vi "Create Agent Refnum.vi"(7 "session":T1, 8 "error in (no error)":errorcluster, 11 "LIBSSH2_AGENT*":u64 format="%.0x") -> (0 "error out":errorcluster, 3 "agent":T2)   [LabVIEW 2013, in "libssh2.lvlib"]
uses:
  libssh2.lvlib
  Agent Refnum.ctl
  Session Refnum.ctl
  Agent Refnum Data.ctl
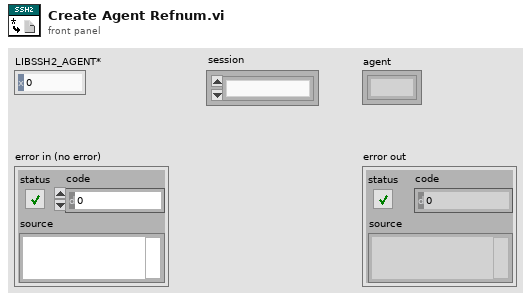
[diagram p1: front panel]
types:
  T1 = typedef "libssh2.lvlib/Session Refnum.ctl" = refnum<k1>
  T2 = typedef "libssh2.lvlib/Agent Refnum.ctl" = refnum<k1>
  T3 = typedef "libssh2.lvlib/Agent Refnum Data.ctl" = cluster{"LIBSSH2_AGENT*":u64, "session":T1}
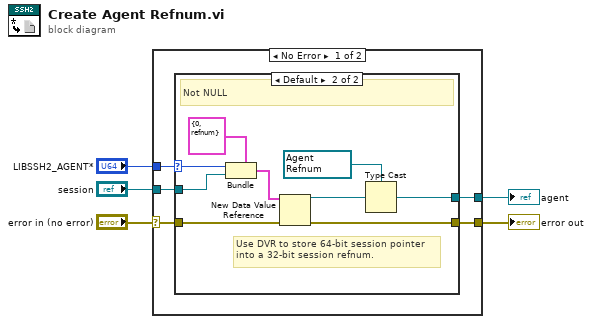
[diagram p0: block diagram]
diagram:
  n1 = case shown="No Error" "error in (no error)" {
    selector: "error in (no error)" -> [w8 w21]
    tunnel: [w10 _] -> w5
    tunnel: "LIBSSH2_AGENT*" -> [w7 _]
    tunnel: [w9 w21] -> w3
    tunnel: "session" -> [w6 _]
    frame No Error {
      n2 = case shown="Default" w7 {
        selector: w7 -> [_ w15]
        tunnel: [_ w18] -> w10
        tunnel: [w11 w17] -> w9
        tunnel: w8 -> [w11 w16]
        tunnel: w6 -> [_ w12]
        frame 0 {
          # "NULL"
        }
        frame Default {
          w19 = T2 refnum items=["Agent"] ("agent")
          # "Use DVR to store 64-bit session pointer\ninto a 32-bit session refnum."
          # "Not NULL"
          n3 = Bundle(cluster=T3 {"LIBSSH2_AGENT*"=0, "session"=refnum} ("agent data"), "LIBSSH2_AGENT*"=w15, "session"=w12) -> (w14:T3)
          n4 = New Data Value Reference(data value=w14, error in=w16) -> (data value reference=w20:refnum<data-value>, error out=w17:errorcluster)
          n5 = Type Cast(type=w19, x=w20) -> (*(type *) &x=w18:T2)
        }
      }
    }
    frame Error {
    }
  }
  "agent" <- w5
  "error out" <- w3
